vi "Success_Evaluator_project.vi"() -> ()   [LabVIEW 2020]
panel:
  in  "Tab Control":enum32{"Page 1", "Page 2"}(tab)
  in  "name":string[](array[string])
  out "Success >=60%":bool[](array[boolean])
  in  "Astronomtic":dbl[](array[numeric])
  in  "Structure":dbl[](array[numeric])
  in  "Orbit":dbl[](array[numeric])
  in  "aviation":dbl[](array[numeric])
  # "Subject"
  # "Student Name"
  # "Success or Failure"
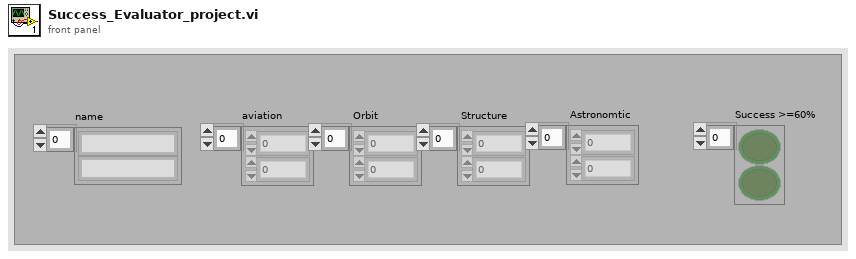
[diagram p1: front panel]
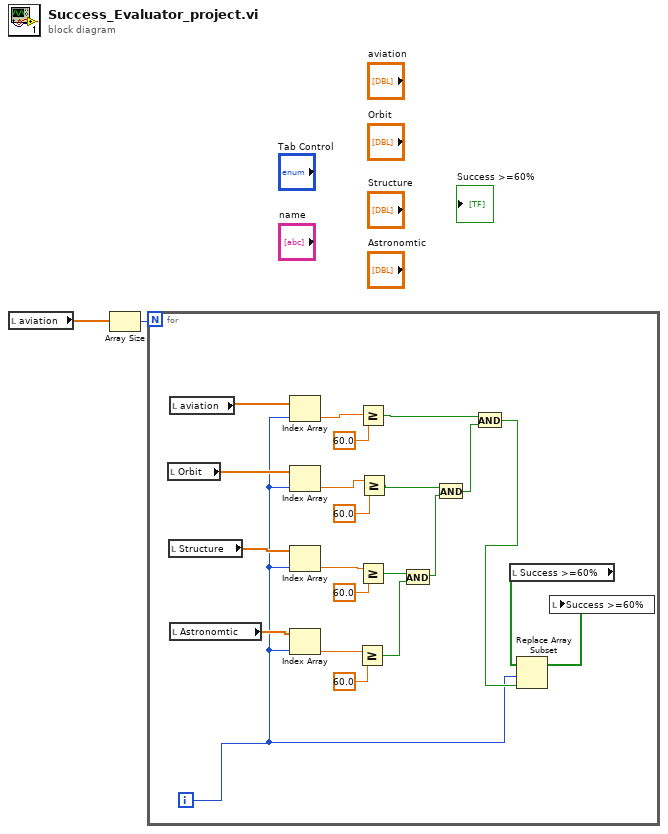
[diagram p0: block diagram]
diagram:
  n1 = local read "aviation"() -> (w2:dbl[])
  n2 = Array Size(array=w2) -> (size(s)=w1:i32)
  n3 = for {
    N: w1 -> [_]
    i -> [w3]
    n4 = local read "Orbit"() -> (w23:dbl[])
    n5 = local read "Structure"() -> (w22:dbl[])
    n6 = local read "aviation"() -> (w24:dbl[])
    n7 = local read "Astronomtic"() -> (w21:dbl[])
    n8 = Index Array(array=w24, index=w3) -> (element=w15:dbl)
    n9 = Index Array(array=w23, index=w3) -> (element=w11:dbl)
    n10 = Index Array(array=w22, index=w3) -> (element=w9:dbl)
    n11 = Index Array(array=w21, index=w3) -> (element=w6:dbl)
    n12 = Greater Or Equal?(x=w6, y=60.0) -> (x >= y?=w4:bool)
    n13 = Greater Or Equal?(x=w15, y=60.0) -> (x >= y?=w13:bool)
    n14 = Greater Or Equal?(x=w9, y=60.0) -> (x >= y?=w7:bool)
    n15 = Greater Or Equal?(x=w11, y=60.0) -> (x >= y?=w12:bool)
    n16 = And(x=w7, y=w4) -> (x .and. y?=w20:bool)
    n17 = And(x=w12, y=w20) -> (x .and. y?=w19:bool)
    n18 = And(x=w13, y=w19) -> (x .and. y?=w16:bool)
    n19 = local read "Success >=60%"() -> (w18:bool[])
    n20 = Replace Array Subset(array=w18, new element=w16, index=w3) -> (w17:bool[])
    n21 = local write "Success >=60%"(w17) -> ()
  }
